vi "AO_WriteData.vi"(7 "data":dbl[](array[numeric]), 8 "error IO":errorcluster, 9 "count":i32, 11 "Task ID":u32) -> (0 "error out":errorcluster, 2 "remaining count":i32, 3 "Task ID":u32)   [LabVIEW 2015]
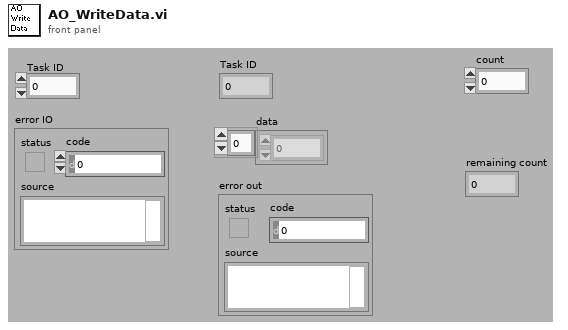
[diagram p1: front panel]
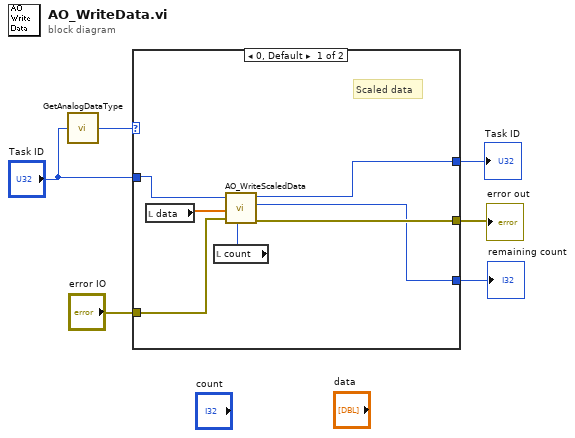
[diagram p0: block diagram]
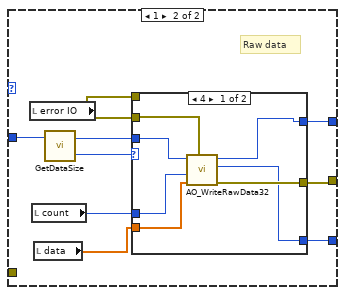
[diagram p2: hidden frame]
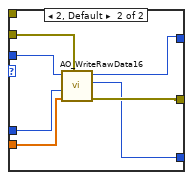
[diagram p3: hidden frame]
diagram:
  n1 = call "GetAnalogDataType.vi"("Task ID"="Task ID") -> ("return type"=w6:i32)
  n2 = case shown="0, Default" w6 {
    tunnel: "Task ID" -> [w12 w22]
    tunnel: "error IO" -> [w11 _]
    tunnel: [w10 w16] -> w3
    tunnel: [w9 w17] -> w2
    tunnel: [w7 w14] -> w1
    frame 0, Default {
      # "Scaled data"
      n3 = local read "data"() -> (w8:dbl[])
      n4 = local read "count"() -> (w13:i32)
      n5 = call "AO_WriteScaledData.vi"("Task ID"=w12, "data"=w8, "error in (no error)"=w11, "count"=w13) -> ("Task ID"=w10:u32, "remaining count"=w7:i32, "error out"=w9:errorcluster)  [unwired: 2 out]
    }
    frame 1 {
      # "Raw data"
      n6 = local read "error IO"() -> (w15:errorcluster)
      n7 = local read "count"() -> (w19:i32)
      n8 = local read "data"() -> (w18:dbl[])
      n9 = call "GetDataSize.vi"("Task ID"=w22) -> ("return type"=w21:i32, "Task ID"=w20:u32)  [unwired: 1 out]
      n10 = case shown="4" w21 {
        tunnel: w20 -> [w28 w36]
        tunnel: w19 -> [w27 w35]
        tunnel: w18 -> [w26 w34]
        tunnel: [w24 w32] -> w17
        tunnel: [w25 w33] -> w16
        tunnel: w15 -> [_ _]
        tunnel: w15 -> [w29 w31]
        tunnel: [w23 w30] -> w14
        frame 4 {
          n11 = call "AO_WriteRawData32.vi"("error in (no error)"=w29, "data"=w26, "count"=w27, "Task ID"=w28) -> ("error out"=w24:errorcluster, "remaining count"=w23:i32, "Task ID"=w25:u32)  [unwired: 1 in, 1 out]
        }
        frame 2, Default {
          n12 = call "AO_WriteRawData16.vi"("error in (no error)"=w31, "data"=w34, "count"=w35, "Task ID"=w36) -> ("error out"=w32:errorcluster, "remaining count"=w30:i32, "Task ID"=w33:u32)  [unwired: 1 in, 1 out]
        }
      }
    }
  }
  "Task ID" <- w3
  "error out" <- w2
  "remaining count" <- w1
